vi "AuxSolve.vi"(0 "Variable Data in":T1, 1 "Array Parsed Expression in":T2[](array[typedef]), 3 "error in (no error)":errorcluster, 4 "VirtualMapping":u16[][](array[numeric])) -> (7 "Variable Data Out":T1, 8 "Array Parsed Expression Out":T2[](array[typedef]), 10 "error out":errorcluster)   [LabVIEW 2014, in "MathProg.lvlib"]
doc: "Calcula solo las medidas auxiliares."
uses:
  MathProg.lvlib
  TypeDefs/ParsedExpression.ctl
  TypeDefs/typeMed.ctl
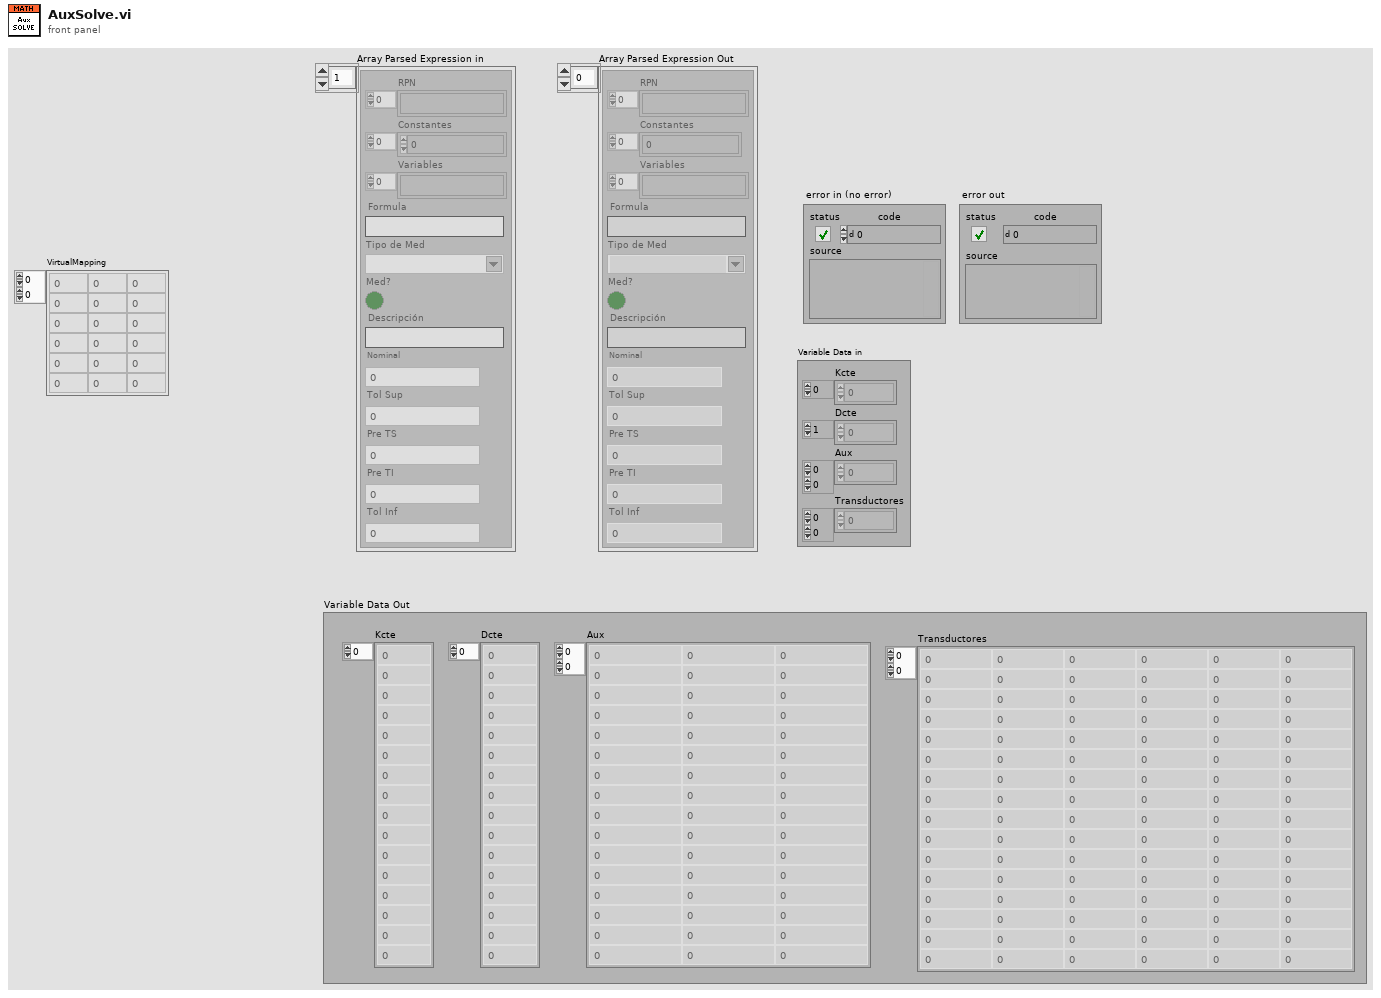
[diagram p1: front panel]
types:
  T1 = cluster{"Kcte":sgl[], "Dcte":sgl[], "Aux":sgl[][], "Transductores":sgl[][]}
  T2 = typedef "MathProg.lvlib/ParsedExpression.ctl" = cluster{"RPN ":string[], "Constantes":sgl[], "Variables":string[], "Formula":string, "Tipo de Med":T3, "Med?":bool, "Descripción":string, "Nominal":sgl, "Tol Sup":sgl, "Pre TS":sgl, "Pre TI":sgl, "Tol Inf":sgl}
  T3 = typedef "MathProg.lvlib/typeMed.ctl" = string
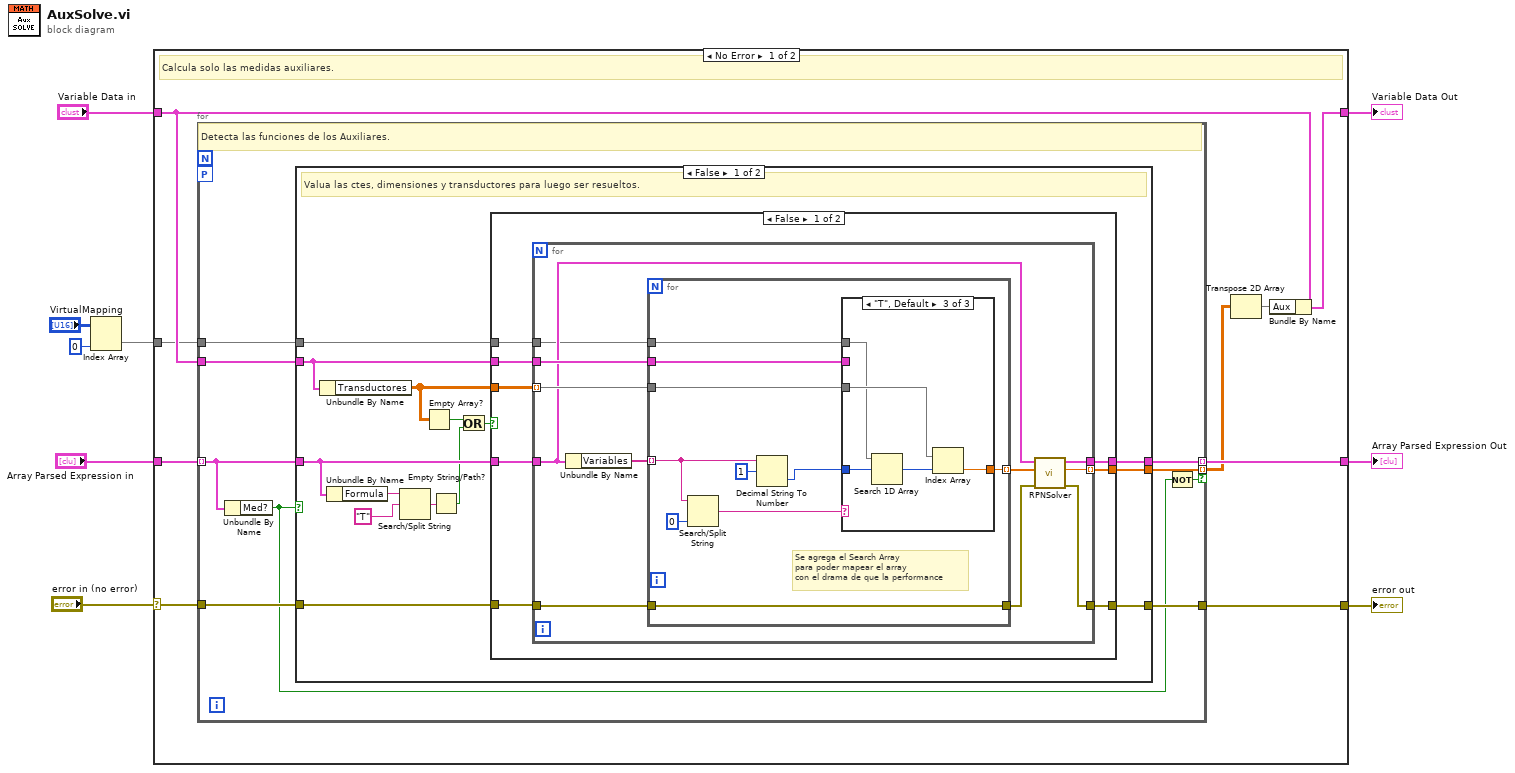
[diagram p0: block diagram]
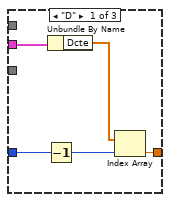
[diagram p2: hidden frame]
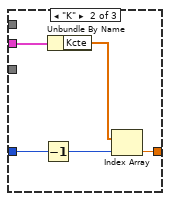
[diagram p3: hidden frame]
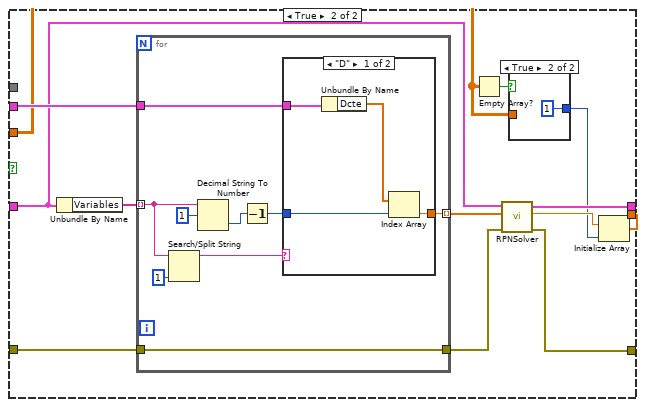
[diagram p4: hidden frame]
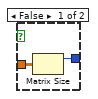
[diagram p5: hidden frame]
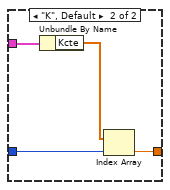
[diagram p6: hidden frame]
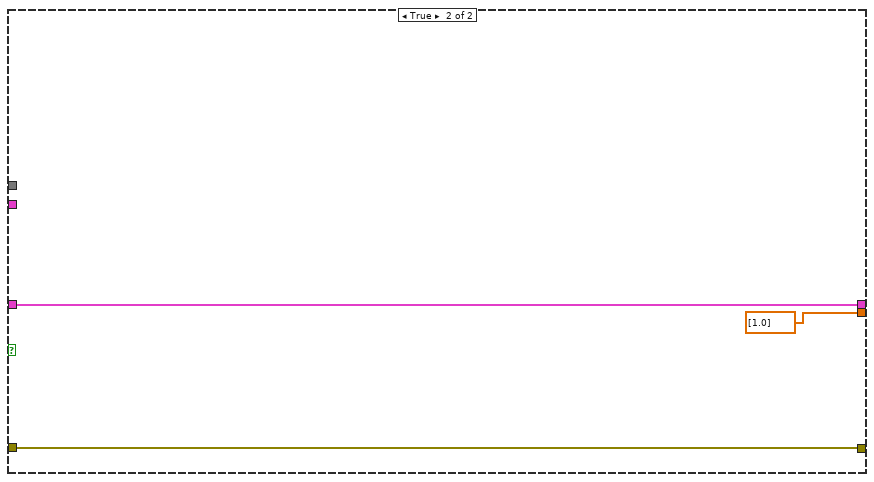
[diagram p7: hidden frame]
diagram:
  n1 = Index Array(array="VirtualMapping", index (col)=0 ("disabled index (col)")) -> (element=w2:u16[])  [unwired: 1 in]
  n2 = case shown="No Error" "error in (no error)" {
    selector: "error in (no error)" -> [w17 w122]
    tunnel: [w18 w122] -> w9
    tunnel: "Variable Data in" -> [w11 w124]
    tunnel: [w16 w123] -> w7
    tunnel: [w15 w124] -> w6
    tunnel: "Array Parsed Expression in" -> [w12 w123]
    tunnel: w2 -> [w10 _]
    frame No Error {
      # "Calcula solo las medidas auxiliares."
      n3 = for {
        tunnel: w12 -> [w27] mode=indexing
        tunnel: w11 -> [w22]
        tunnel: [w26] -> w13 mode=indexing if=w21
        tunnel: [w23] -> w16 mode=indexing
        tunnel: [w25] -> w18
        tunnel: w17 -> [w24]
        workers-P: _ -> [_]
        tunnel: w10 -> [w19]
        # "Detecta las funciones de los Auxiliares."
        n4 = Unbundle By Name(w27) -> ("Med?"=w20:bool)
        n5 = case shown="False" w20 {
          tunnel: w27 -> [w35 w120]
          tunnel: [w41 sgl[] [1.0]] -> w26
          tunnel: [w39 w121] -> w25
          tunnel: w24 -> [w38 w121]
          tunnel: [w40 w120] -> w23
          tunnel: w22 -> [w37 _]
          tunnel: w19 -> [w28 _]
          frame False {
            # "Valua las ctes, dimensiones y transductores para luego ser resueltos."
            n6 = Unbundle By Name(w37) -> ("Transductores"=w36:sgl[][])
            n7 = Unbundle By Name(w35) -> ("Formula"=w34:string)
            n8 = Search/Split String(string=w34, search string/char (-)="T") -> (match + rest of string=w32:string)  [unwired: 1 in, 2 out]
            n9 = Empty Array?(array=w36) -> (empty?=w31:bool)
            n10 = Empty String/Path?(string/path=w32) -> (empty?=w29:bool)
            n11 = Or(x=w31, y=w29) -> (x .or. y?=w30:bool)
            n12 = case shown="False" w30 {
              tunnel: [w49 w90] -> w41
              tunnel: w35 -> [w48 w94]
              tunnel: [w47 w92] -> w40
              tunnel: [w46 w93] -> w39
              tunnel: w38 -> [w45 w95]
              tunnel: w37 -> [w44 w96]
              tunnel: w36 -> [w43 w86]
              tunnel: w28 -> [w42 _]
              frame False {
                n13 = for {
                  tunnel: [w56] -> w49 mode=indexing
                  tunnel: w48 -> [w51]
                  tunnel: [w55] -> w47
                  tunnel: w44 -> [w57]
                  tunnel: w43 -> [w58] mode=indexing
                  tunnel: w45 -> [w59]
                  tunnel: [w52] -> w46
                  tunnel: w42 -> [w50]
                  n14 = Unbundle By Name(w51) -> ("Variables"=w60:string[])
                  n15 = for {
                    tunnel: w60 -> [w65] mode=indexing
                    tunnel: w59 -> [w67]
                    tunnel: w58 -> [w70]
                    tunnel: w57 -> [w69]
                    tunnel: [w68] -> w54 mode=indexing
                    tunnel: [w67] -> w53
                    tunnel: w50 -> [w61]
                    # "Se agrega el Search Array\npara poder mapear el array\ncon el drama de que la performance"
                    n16 = Search/Split String(string=w65, offset (0)=0) -> (match + rest of string=w63:string)  [unwired: 1 in, 2 out]
                    n17 = Decimal String To Number(string=w65, offset=1) -> (number=w62:i32)  [unwired: 1 in, 1 out]
                    n18 = case shown="\"T\", Default" w63 {
                      tunnel: [w73 w80 w85] -> w68
                      tunnel: w70 -> [_ _ w84]
                      tunnel: w69 -> [w74 w79 _]
                      tunnel: w62 -> [w72 w77 w82]
                      tunnel: w61 -> [_ _ w83]
                      frame "D" {
                        n19 = Decrement(x=w72) -> (x-1=w71:i32)
                        n20 = Unbundle By Name(w74) -> ("Dcte"=w75:sgl[])
                        n21 = Index Array(array=w75, index=w71) -> (element=w73:sgl)
                      }
                      frame "K" {
                        n22 = Decrement(x=w77) -> (x-1=w76:i32)
                        n23 = Unbundle By Name(w79) -> ("Kcte"=w78:sgl[])
                        n24 = Index Array(array=w78, index=w76) -> (element=w80:sgl)
                      }
                      frame "T", Default {
                        n25 = Search 1D Array(1D array=w83, element=w82) -> (index of element=w81:i32)  [unwired: 1 in]
                        n26 = Index Array(array=w84, index=w81) -> (element=w85:sgl)
                      }
                    }
                  }
                  n27 = call "RPNSolver.vi"("error in"=w53, "Variable Value Array"=w54, "Parsed Expression In"=w51) -> ("error out"=w52:errorcluster, "Numeric"=w56:sgl, "Parsed Expression Out"=w55:T2)  [unwired: 5 in]
                }
              }
              frame True {
                n28 = Unbundle By Name(w94) -> ("Variables"=w97:string[])
                n29 = for {
                  tunnel: w97 -> [w104] mode=indexing
                  tunnel: w95 -> [w108]
                  tunnel: w96 -> [w110]
                  tunnel: [w109] -> w91 mode=indexing
                  tunnel: [w108] -> w98
                  n30 = Search/Split String(string=w104, offset (0)=1 ("length (rest)")) -> (substring before match=w103:string)  [unwired: 1 in, 2 out]
                  n31 = Decimal String To Number(string=w104, offset=1) -> (number=w106:i32)  [unwired: 1 in, 1 out]
                  n32 = Decrement(x=w106) -> (x-1=w105:i32)
                  n33 = case shown="\"D\"" w103 {
                    tunnel: [w112 w115] -> w109
                    tunnel: w110 -> [w113 w118]
                    tunnel: w105 -> [w111 w116]
                    frame "D" {
                      n34 = Unbundle By Name(w113) -> ("Dcte"=w114:sgl[])
                      n35 = Index Array(array=w114, index=w111) -> (element=w112:sgl)
                    }
                    frame "K", Default {
                      n36 = Unbundle By Name(w118) -> ("Kcte"=w117:sgl[])
                      n37 = Index Array(array=w117, index=w116) -> (element=w115:sgl)
                    }
                  }
                }
                n38 = Empty Array?(array=w86) -> (empty?=w88:bool)
                n39 = call "RPNSolver.vi"("error in"=w98, "Variable Value Array"=w91, "Parsed Expression In"=w94) -> ("error out"=w93:errorcluster, "Numeric"=w89:sgl, "Parsed Expression Out"=w92:T2)  [unwired: 5 in]
                n40 = case shown="True" w88 {
                  tunnel: [w99 1 ("number of columns")] -> w87
                  tunnel: w86 -> [w100 _]
                  frame False {
                    n41 = Matrix Size(0:w100) -> (1:w99:i32)  [unwired: 1 out]
                  }
                  frame True {
                  }
                }
                n42 = Initialize Array(w89, w87) -> (w90:sgl[])
              }
            }
          }
          frame True {
          }
        }
        n43 = Not(x=w20) -> (.not. x?=w21:bool)
      }
      n44 = Transpose 2D Array(2D array=w13) -> (transposed array=w14:sgl[][])
      n45 = Bundle By Name(cluster=w11, "Aux"=w14) -> (w15:T1)
    }
    frame Error {
    }
  }
  "error out" <- w9
  "Array Parsed Expression Out" <- w7
  "Variable Data Out" <- w6
